vi "Open UDP Port.vi"(7 "net address":u32, 8 "error in (no error)":errorcluster, 9 "timeout ms (25000)":i32, 10 "service name":string, 11 "UDPPort":u16) -> (0 "error out":errorcluster, 2 "UsedPort":u16, 3 "UDP Network Connection out":refnum<k16>)   [LabVIEW 2015, in "AMC.lvlib"]
uses:
  AMC.lvlib
  Globals.vi
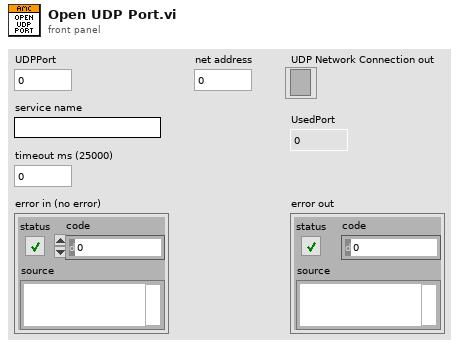
[diagram p1: front panel]
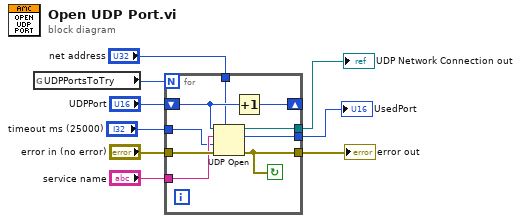
[diagram p0: block diagram]
diagram:
  n1 = global read "Globals.vi" "UDPPortsToTry"() -> (w1:i32)
  n2 = for {
    N: w1 -> [_]
    tunnel: "service name" -> [w16]
    tunnel: [w15] -> w4
    tunnel: "error in (no error)" -> [w17]
    tunnel: [w14] -> w9
    tunnel: [w18] -> w8
    shift-right: [w12] -> _
    shift-left: "UDPPort" -> [w13]
    tunnel: "timeout ms (25000)" -> [w11]
    tunnel: "net address" -> [w10]
    stop <- w14 continue-if-true
    n3 = UDP Open(7:w10, 8:w17, 9:w11, 10:w16, 11:w13) -> (port=w15:refnum<k16>, 0:w14:errorcluster, 2:w18:u16)
    n4 = Increment(x=w13) -> (x+1=w12:u16)
  }
  "error out" <- w9
  "UsedPort" <- w8
  "UDP Network Connection out" <- w4
